vi "Select menu measurements.vi"(8 "error in (no error)":errorcluster, 10 "Measurements":string[](array[string]), 11 "Common Measurements Interface in":refnum<class "Common Measurements Interface.lvclass">) -> (0 "error out":errorcluster, 3 "Common Measurements Interface out":refnum<class "Common Measurements Interface.lvclass">)   [LabVIEW 2015, in "Common Measurements Interface.lvclass"]
uses:
  Common Measurements Interface.lvclass
  Common Measurements Interface.lvclass/Common Measurements Interface.ctl
  Queued Listbox/Queued Listbox.xctl
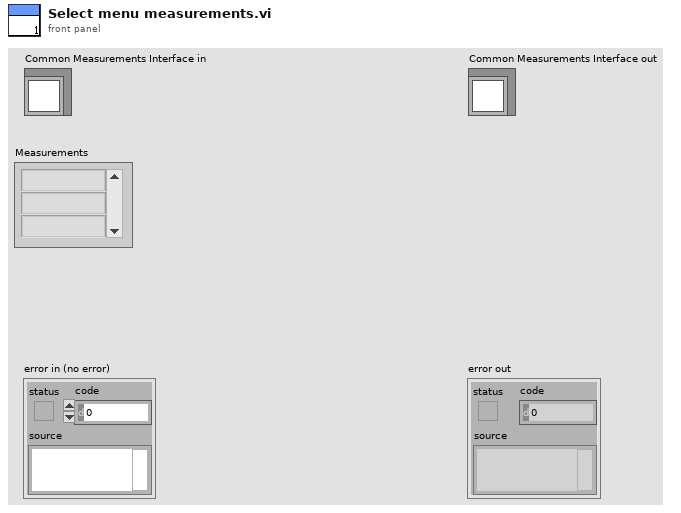
[diagram p1: front panel]
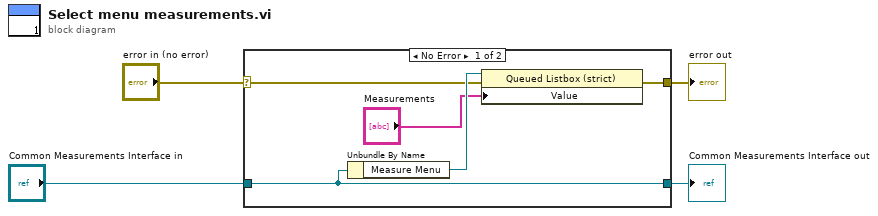
[diagram p0: block diagram]
diagram:
  n1 = case shown="No Error" "error in (no error)" {
    selector: "error in (no error)" -> [w6 w11]
    tunnel: [w5 w11] -> w3
    tunnel: [w9 w10] -> w1
    tunnel: "Common Measurements Interface in" -> [w9 w10]
    frame No Error {
      n2 = Unbundle By Name(w9) -> ("Measure Menu"=w8:refnum<vi>)
      n3 = property class="Queued Listbox (strict)"(reference=w8, error in=w6, "Value"="Measurements") -> (error out=w5:errorcluster)  [unwired: 1 out]
    }
    frame Error {
    }
  }
  "error out" <- w3
  "Common Measurements Interface out" <- w1
